vi "Averaging.vi"(8 "error in (no error)":errorcluster, 10 "Averaging Number (8:256)":u32(ring)=8 items=["1", "2", "4", "8", "16", "32", "64", "128", "256"], 11 "VISA resource name":refnum<visa-resource-name>) -> (0 "error out":errorcluster, 3 "VISA resource name out":refnum<visa-resource-name>)   [LabVIEW 2017, in "Agilent 4194.lvlib"]
doc: "This function specifies the averaging number."
uses:
  PiezoST/Agilent 4194/Agilent 4194.lvlib
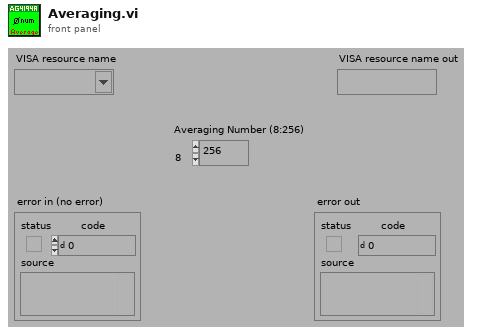
[diagram p1: front panel]
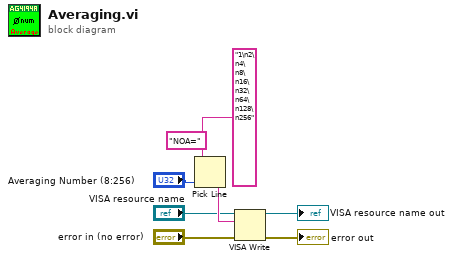
[diagram p0: block diagram]
diagram:
  n1 = Pick Line(string ("")="NOA=", multi-line string="1\n2\n4\n8\n16\n32\n64\n128\n256", line index="Averaging Number (8:256)") -> (output string=w6:string)
  n2 = VISA Write(VISA resource name="VISA resource name", write buffer=w6, error in (no error)="error in (no error)") -> (VISA resource name out=→"VISA resource name out":refnum<visa-resource-name>, error out=→"error out":errorcluster)  [unwired: 1 out]
